vi "WSD Request Compose.vi"(7 "Checksum used":bool=TRUE, 9 "Data":i16[](array[numeric]) format="%x", 10 "D-register number":u32=1, 11 "Address":u8=1) -> (3 "Request":string, 4 "Command":string="WSD")   [LabVIEW 2015, in "Samwontech TEMP2xxx.lvlib"]
uses:
  Samwontech TEMP2xxx.lvlib
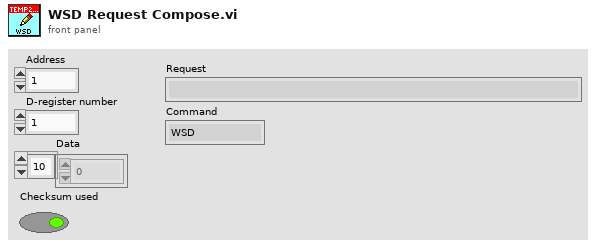
[diagram p1: front panel]
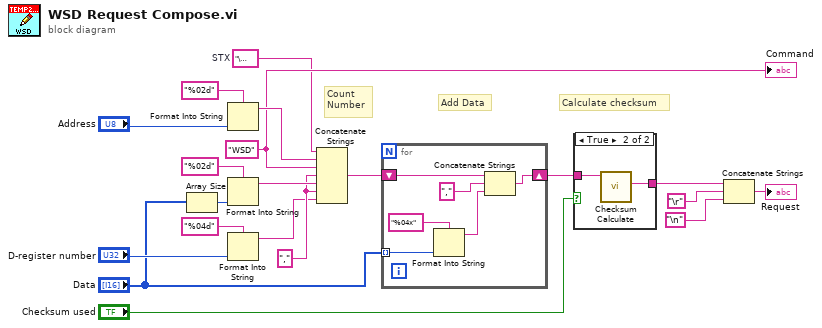
[diagram p0: block diagram]
diagram:
  w16 = "," ("format string")
  w18 = "WSD" ("format string")
  w9 = "\u0002"  # STX
  # "Add Data"
  # "Count\nNumber"
  # "Calculate checksum"
  n1 = Array Size(array="Data") -> (size(s)=w7:i32)
  n2 = Format Into String(format string="%02d", "Address") -> (resulting string=w19:string)  [unwired: 2 in, 1 out]
  n3 = Format Into String(format string="%02d", w7) -> (resulting string=w17:string)  [unwired: 2 in, 1 out]
  n4 = Format Into String(format string="%04d", "D-register number") -> (resulting string=w13:string)  [unwired: 2 in, 1 out]
  n5 = Concatenate Strings(w9, w19, w18, w16, w17, w16, w13) -> (w3:string)
  n6 = for {
    shift-right: [w21] -> w1
    shift-left: w3 -> [w23]
    tunnel: "Data" -> [w24] mode=indexing
    n7 = Format Into String(format string="%04x", w24) -> (resulting string=w22:string)  [unwired: 2 in, 1 out]
    n8 = Concatenate Strings(w23, "," ("format string"), w22) -> (w21:string)
  }
  n9 = case shown="True" "Checksum used" {
    tunnel: w1 -> [w27 w29]
    tunnel: [w27 w28] -> w8
    frame False {
    }
    frame True {
      n10 = call "Checksum Calculate.vi"("Command in"=w29) -> ("Command out (with checksum)"=w28:string)  [unwired: 7 in, 3 out]
    }
  }
  n11 = Concatenate Strings(w8, "\r", "\n") -> (→"Request":string)
  "Command" <- w18
